vi "01-ConversaoCelsiusParaFahrenheit.vi"(1 "Deg C":dbl) -> (0 "Deg F":dbl)   [LabVIEW 2014]
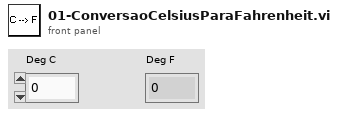
[diagram p1: front panel]
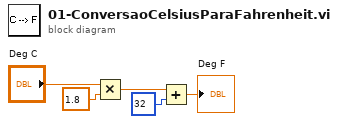
[diagram p0: block diagram]
diagram:
  n1 = Multiply(x="Deg C", y=1.8) -> (x*y=w3:dbl)
  n2 = Add(x=w3, y=32) -> (x+y=→"Deg F":dbl)
